vi "主程序-复材超声C扫缺陷分析评定软件.vi"() -> ()   [LabVIEW 2018]
doc: "使用该模板构建用户界面事件处理设计模式。将模板应用于对话框及其它用户界面。用户也可创建并执行VI可按照与用户界面事件相同方式处理的用户定义事件。"
uses:
  <vilib>/Utility/NIReport.llb/Report Type.ctl
  <vilib>/addons/_office/_exclsub.llb/font.ctl
  <vilib>/Utility/NIReport.llb/HTML Report Image Alignment.ctl
  <vilib>/Utility/NIReport.llb/Append Report Text (str wrap).vi
  <vilib>/Utility/NIReport.llb/Append Image to Report (path wrap).vi
  <vilib>/addons/_office/word.llb/Word Easy Table (str).vi
  <vilib>/Utility/NIReport.llb/NI_report.lvclass
  <vilib>/Utility/NIReport.llb/Word/NI_Word.lvclass
  <vilib>/addons/_office/NI_ReportGenerationToolkit.lvlib
  <vilib>/Utility/NIReport.llb/NI_ReportGenerationCore.lvlib
  <vilib>/vision/NI_Vision_Development_Module.lvlib
panel:
  out "框号-报告图中按顺序的值":i32
  out "框号-更新后按顺序的值":i32
  out "XY向分辨率":T1
  out "flag数组":i8[](array[numeric])
  out "字符串":string
  out "图像Y向分辨率（mm/像素）":dbl
  out "图像X向分辨率（mm/像素）":dbl
  out "判定为筋条的长宽比阈值":i32
  out "框号字体大小-":i16
  out "是否需要预处理":u16
  out "计入缺陷的Z值阈值":i32 caption="值"
  out "计入缺陷的面积阈值":i32
  out "报告模式":string
  in  "删除标注":bool caption="定量分析"
  out "缺陷灰度阈值":dbl caption="值"
  out "穿透图原始路径":path
  out "ROImask":T2(plugin-control)
  out "添加的路径":path
  out "连接的字符串 2":string
  out "临界面积百分比值":dbl
  out "临界Z值":i32
  out "标注后的图片路径":path
  out "全部检测结果合并":string[][](table)
  out "全部检测结果":string[][](table)
  out "部位信息":string[](array[string])=["", "34.500000", "32.500000", "1121", "34", "54.955926", "分层类", "不合格", ""]
  in  "完成标注":bool caption="定量分析"
  out "框数":dbl
  out "自定义字体":T3={"Desired Font (Application)"=enum."Application Font", "[User-specified Font]"={"Font Name"="", "Size"=12, "Strikeout?"=FALSE, "Italic?"=FALSE, "Underline?"=FALSE, "Outline?"=FALSE, "Shadow?"=FALSE, "Bold?"=FALSE, "Rotation Angle"=0.0}, "Horizontal Alignment"=0, "Vertical Alignment"=0} {"Horizontal Alignment" items=["Left", "Center", "Right"]; "Vertical Alignment" items=["Bottom", "Top", "Baseline"]}
  out "框组":T4(array[cluster])
  out "质量等级":string
  in  "stop":bool caption="停止"
  in  "导入图像":bool caption="导入图片"
  in  "开始标注":bool caption="定量分析"
  in  "查看评定结果":bool caption="辅助定性分析"
  in  "生成报告":bool caption="生成原始记录"
  in  "控件":enum32{"穿透图"}(tab)
  out "穿透图":T2(plugin-control)
  out "产品规格":cluster{"产品长度（周长）（mm）":dbl, "产品宽度（母线长）（mm）":dbl}
  out "图像分辨率":T1
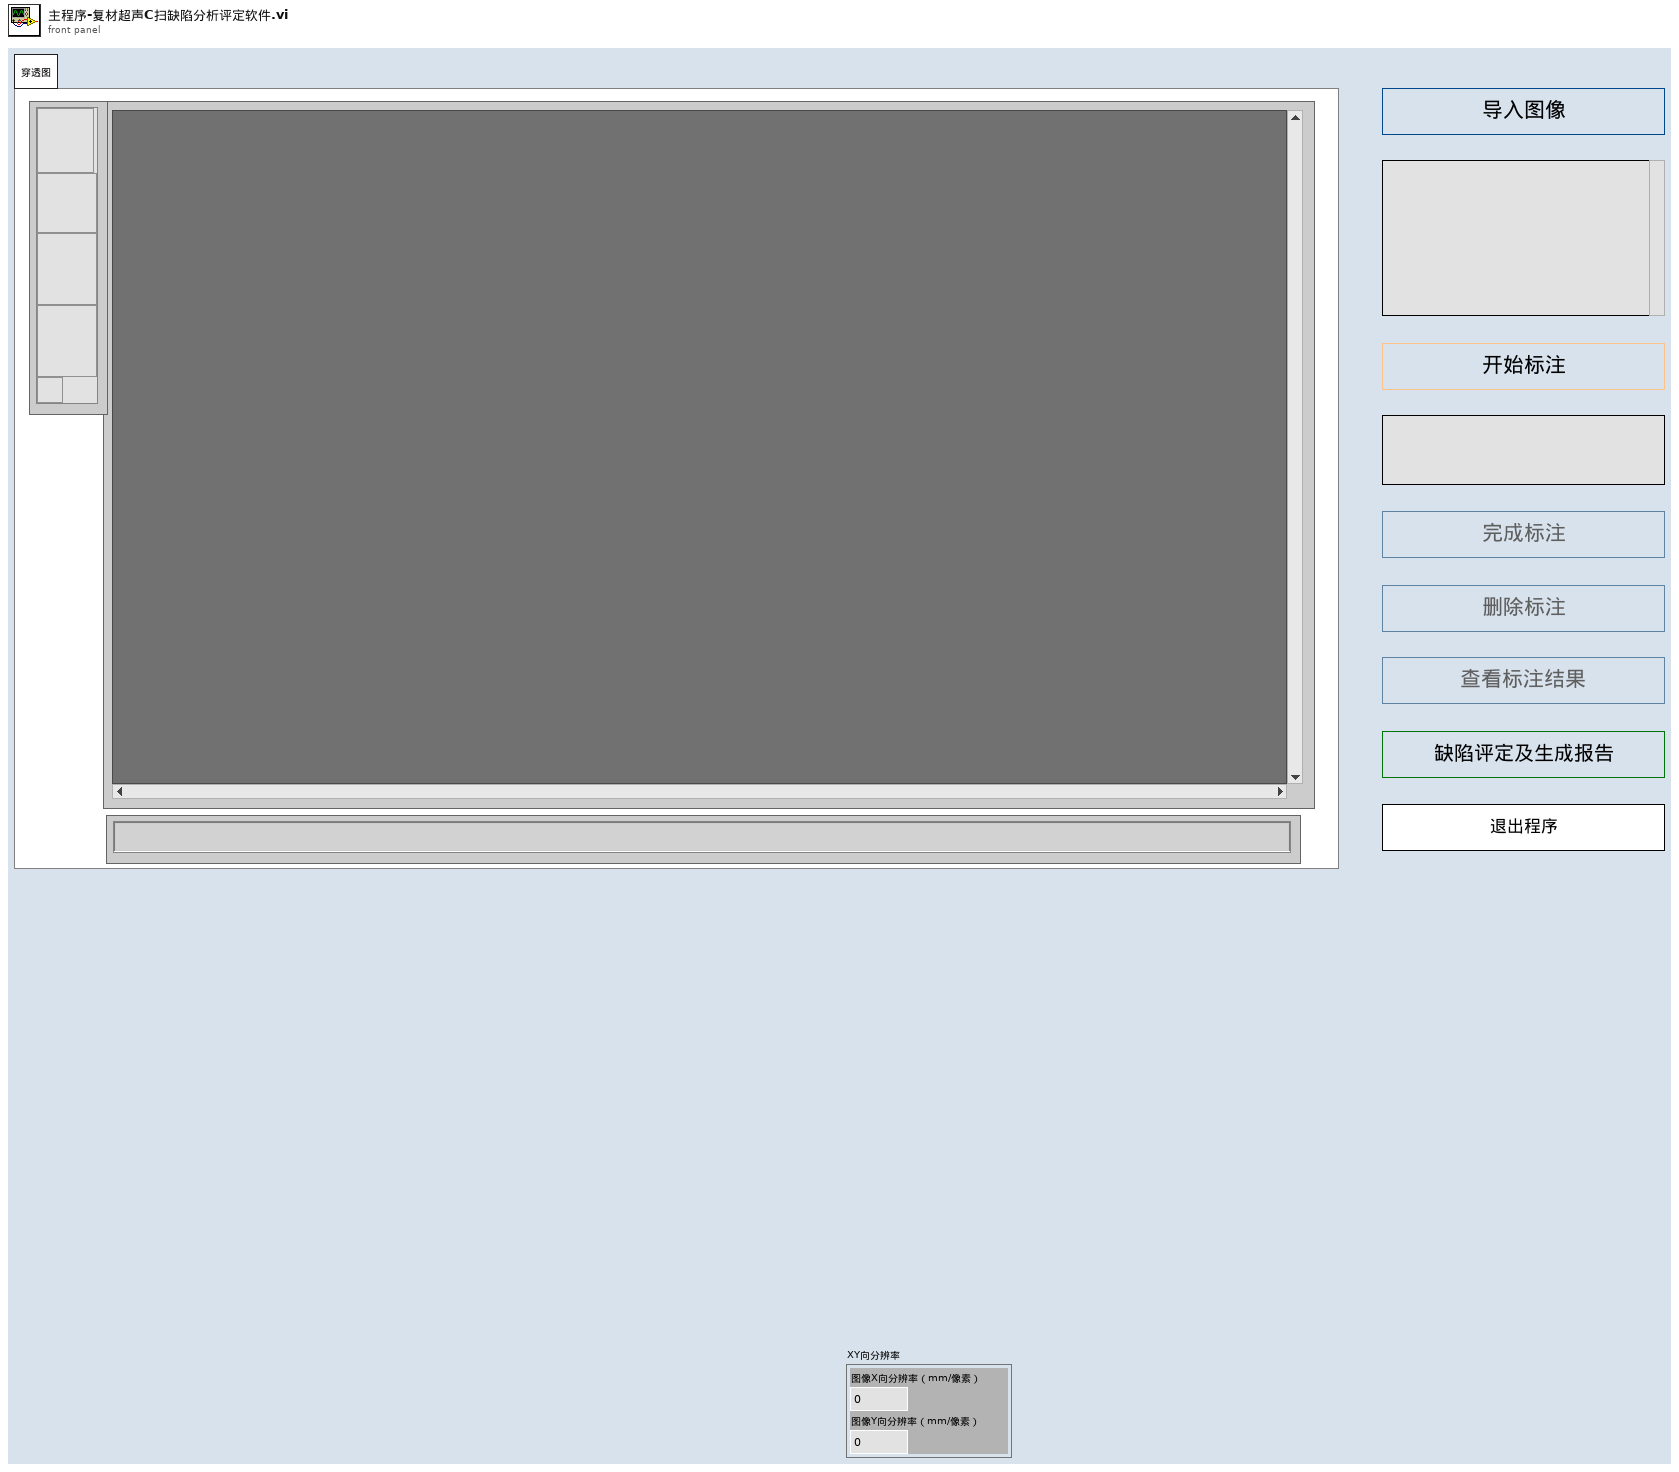
[diagram p1: front panel]
types:
  T1 = cluster{"图像X向分辨率（mm/像素）":dbl, "图像Y向分辨率（mm/像素）":dbl}
  T2 = typedef "IMAQ Image.ctl" = refnum<image>
  T3 = cluster{"Desired Font (Application)":enum16{"User-specified Font", "Application Font", "System Font", "Dialog Font"}, "[User-specified Font]":cluster{"Font Name":string, "Size":i16, "Strikeout?":bool, "Italic?":bool, "Underline?":bool, "Outline?":bool, "Shadow?":bool, "Bold?":bool, "Rotation Angle":dbl}, "Horizontal Alignment":i16, "Vertical Alignment":i16}
  T4 = cluster{"Global Rectangle":i32[], "Contours":cluster{"Contour Type":u32, "ROI Type":u32, "Points":i32[]}[]}[]
  T5 = enum8{"Enabled", "Disabled", "Disabled and Grayed Out"}
  T6 = cluster{"Global Rectangle":i32[], "Contours":cluster{"Contour Type":u32, "ROI Type":u32, "Points":i32[]}[]}
  T7 = cluster{"Zoom Tool":bool, "Selection Tool":bool, "Pan Tool":bool, "Point Tool":bool, "Line Tool":bool, "Rectangle Tool":bool, "Rotated Rectangle Tool":bool, "Polyline Tool":bool, "Polygon Tool":bool, "Freehand Tool":bool, "Closed Freehand Tool":bool, "Ellipse Tool":bool, "Annulus Tool":bool}
  T8 = enum16{"maximized", "minimized", "normal", "no change"}
  T9 = typedef "NI_ReportGenerationCore.lvlib/Report Type.ctl" = enum16{"HTML", "Word", "Excel"}
  T10 = typedef "NI_ReportGenerationCore.lvlib/HTML Report Image Alignment.ctl" = enum16{"(default)", "LEFT", "RIGHT", "TOP", "TEXTTOP", "MIDDLE", "ABSMIDDLE", "BASELINE", "BOTTOM", "ABSBOTTOM"}
  T11 = cluster{"position (Excel)":cluster{"row":i32, "column":i32}, "name (Excel)":string, "bookmark (Word)":string}
  T12 = cluster{"position (excel)":cluster{"row":i32, "column":i32}, "name (excel)":string, "bookmark (word)":string}
  T13 = typedef "NI_ReportGenerationToolkit.lvlib/font.ctl" = cluster{"font name":string, "font size":dbl, "bold":u16, "italic":u16, "underline":u16, "strike through":u16, "font color":u32}
  T14 = typedef "Image Type" = u32
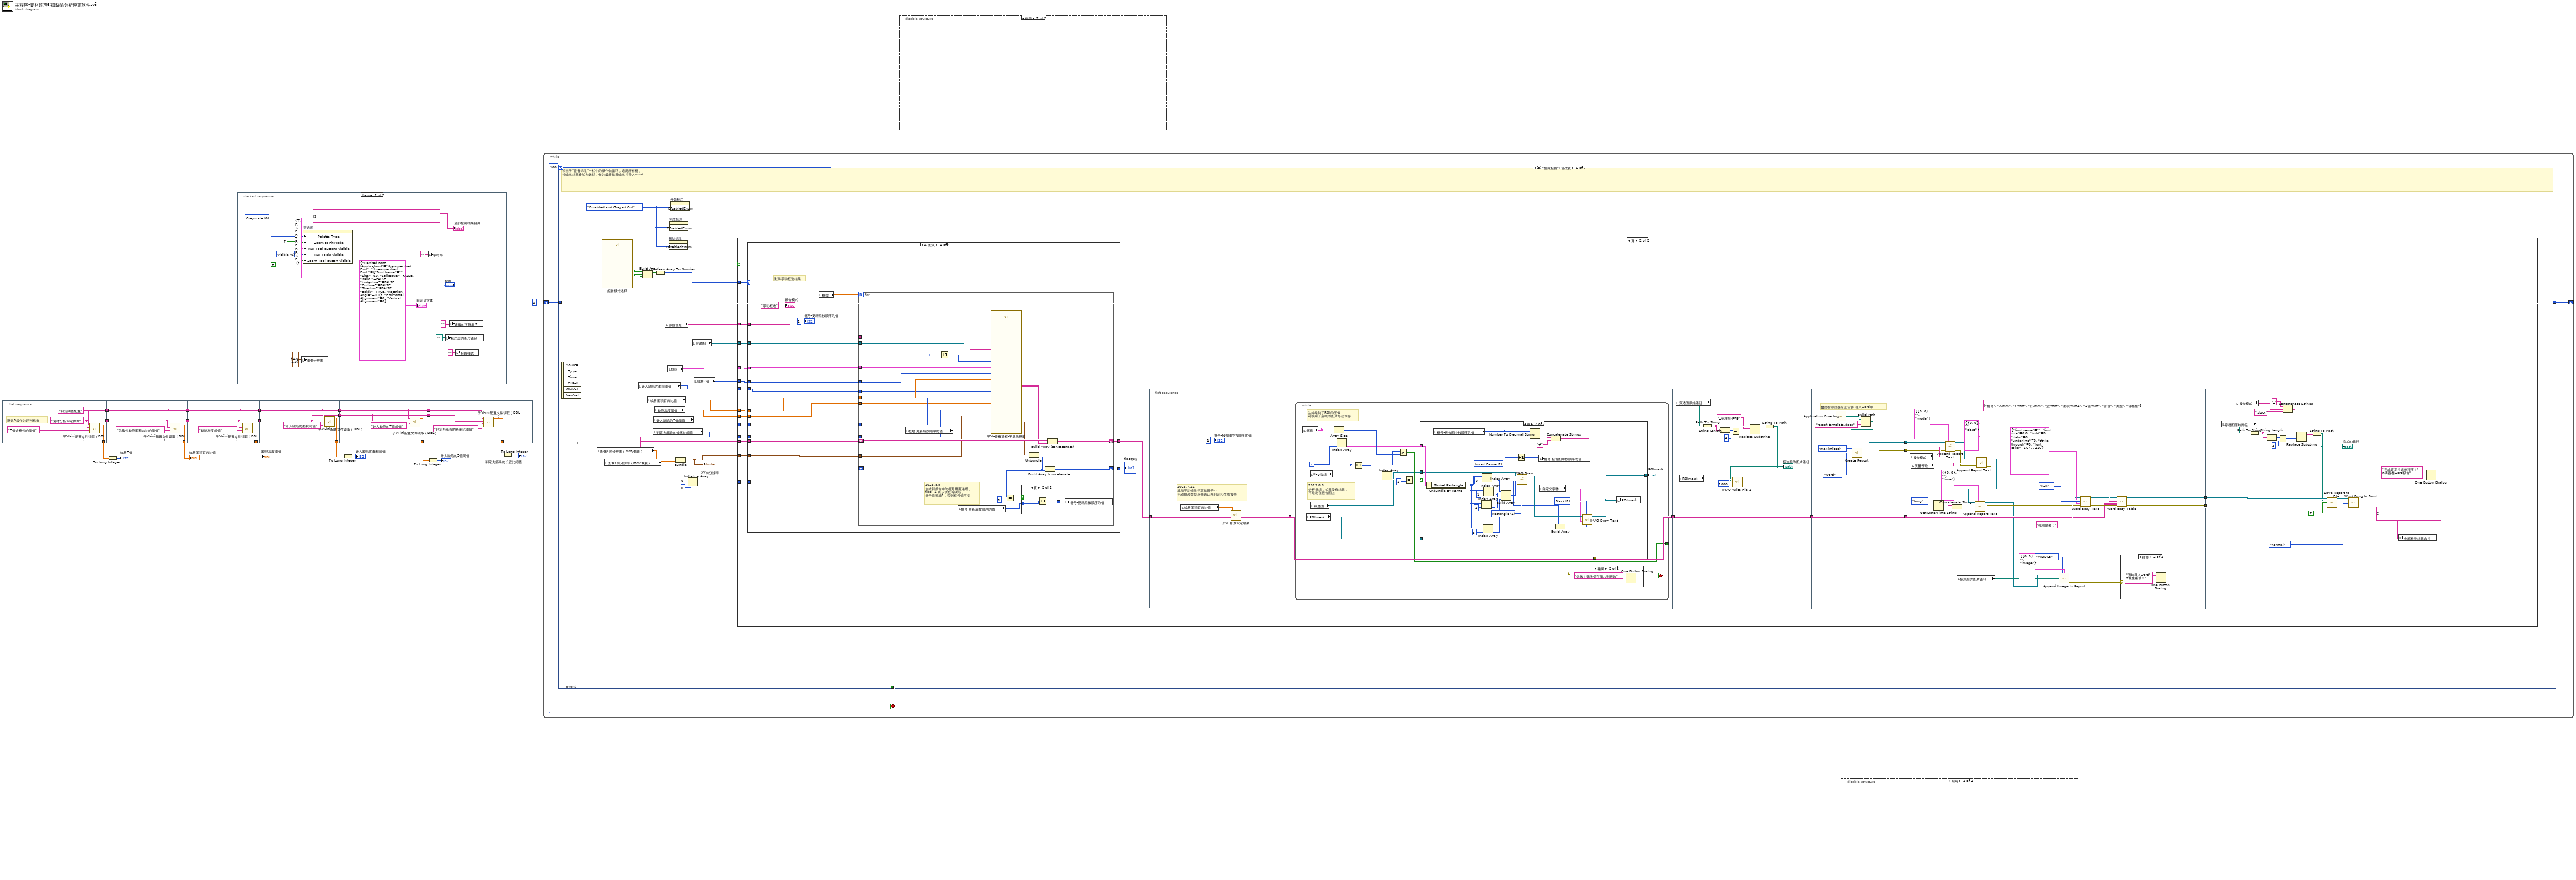
[diagram p0: block diagram]
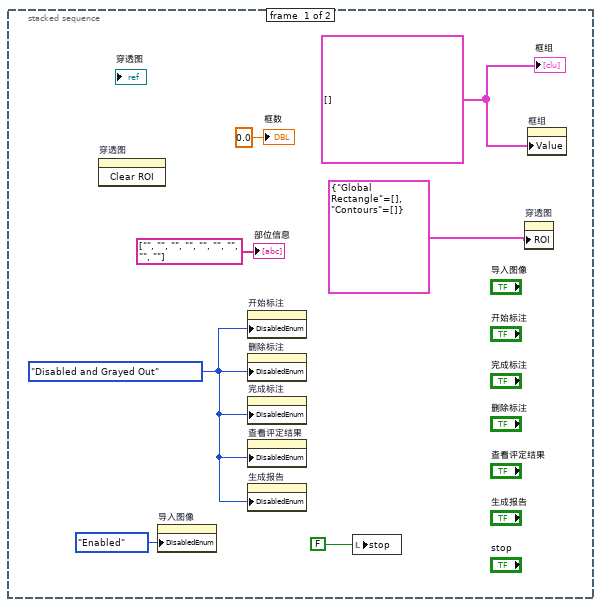
[diagram p3: hidden frame]
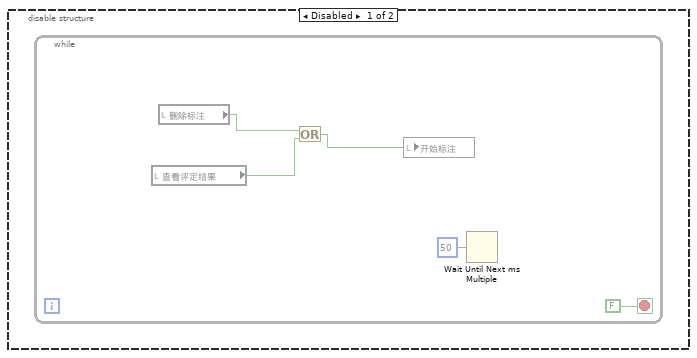
[diagram p4: hidden frame]
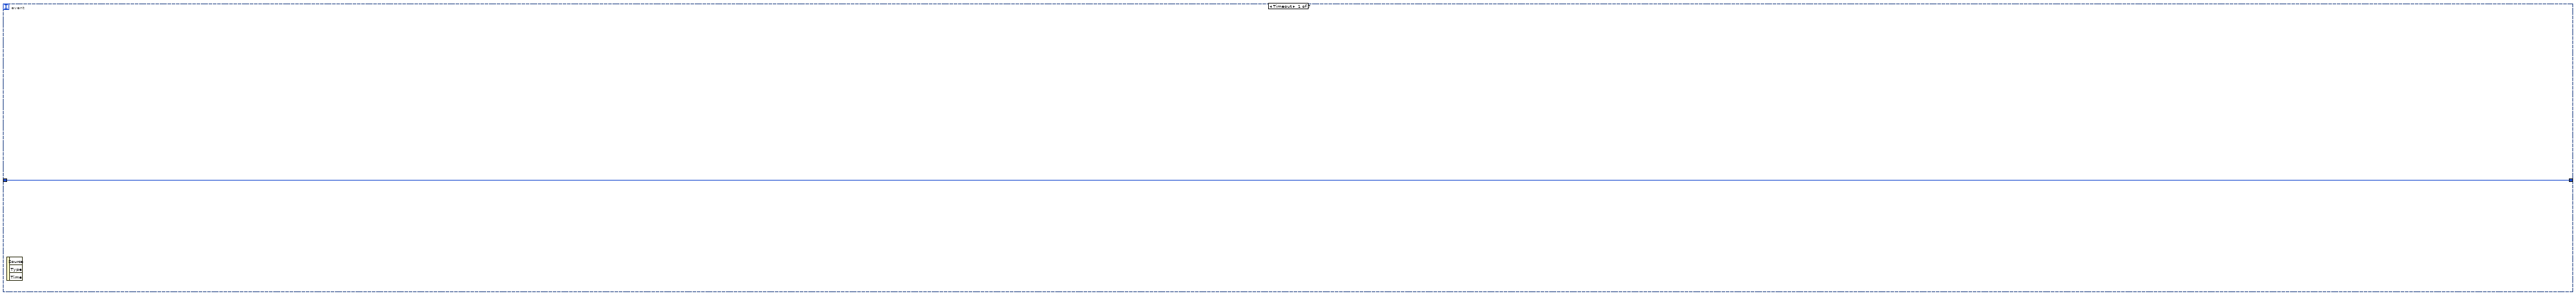
[diagram p5: hidden frame]
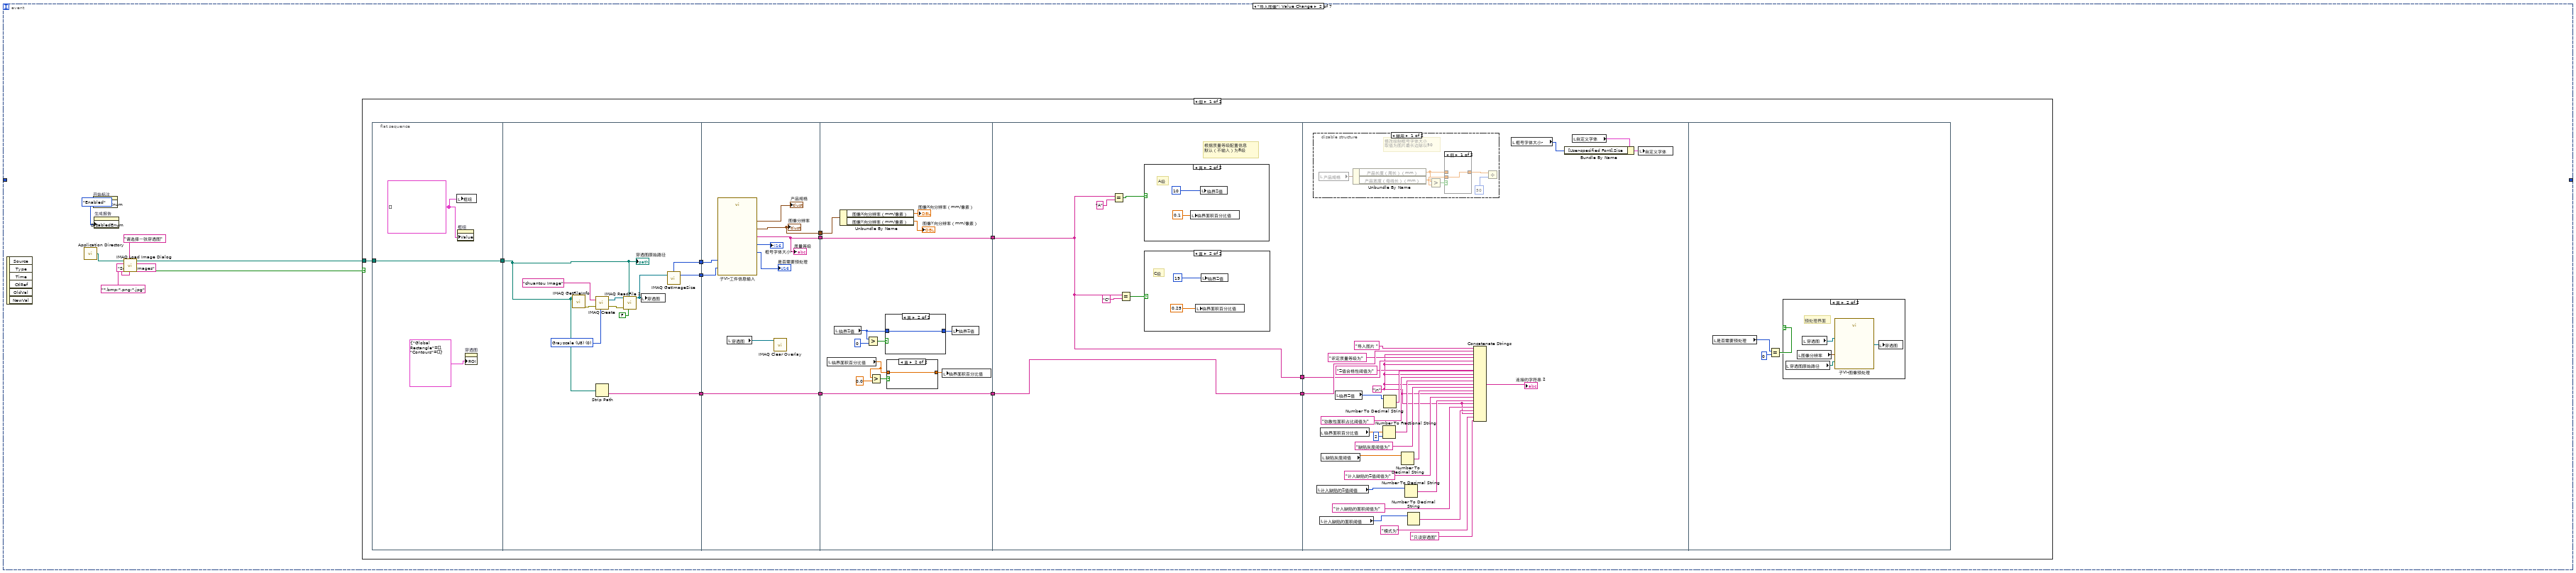
[diagram p6: hidden frame]
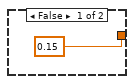
[diagram p7: hidden frame]
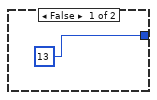
[diagram p8: hidden frame]
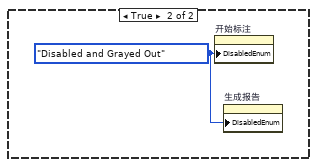
[diagram p14: hidden frame]
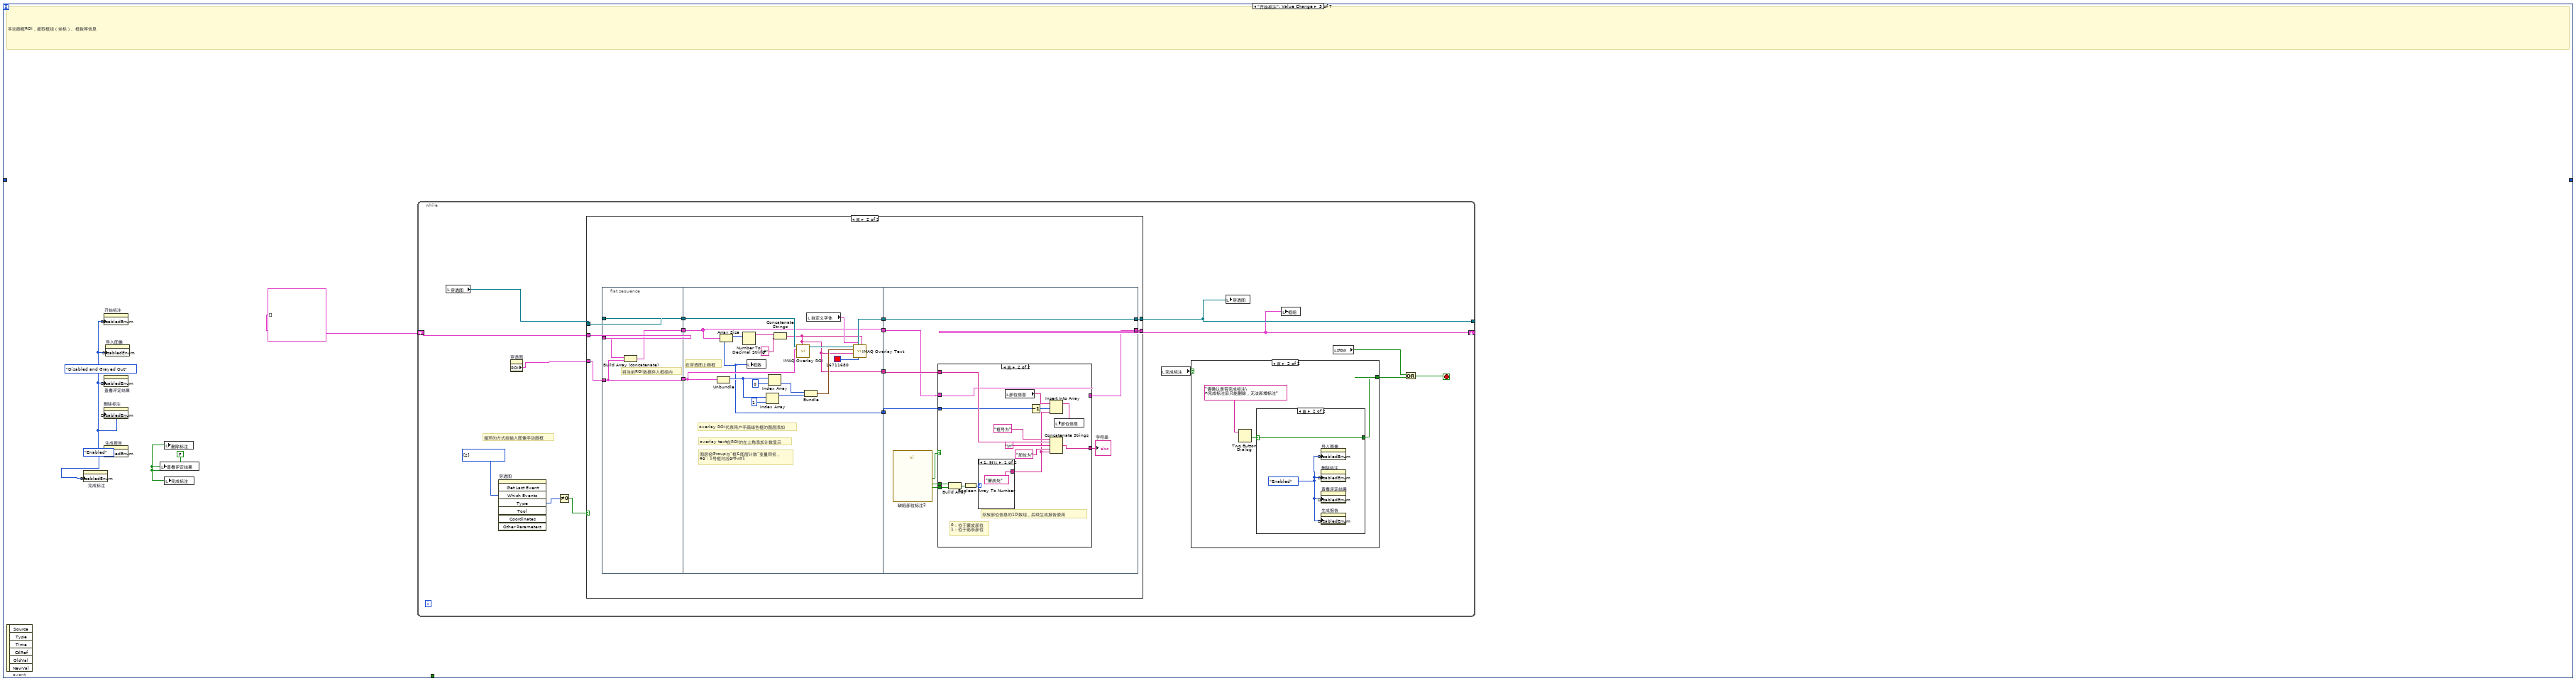
[diagram p15: hidden frame]
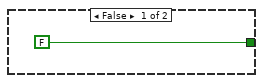
[diagram p16: hidden frame]
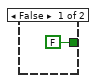
[diagram p17: hidden frame]
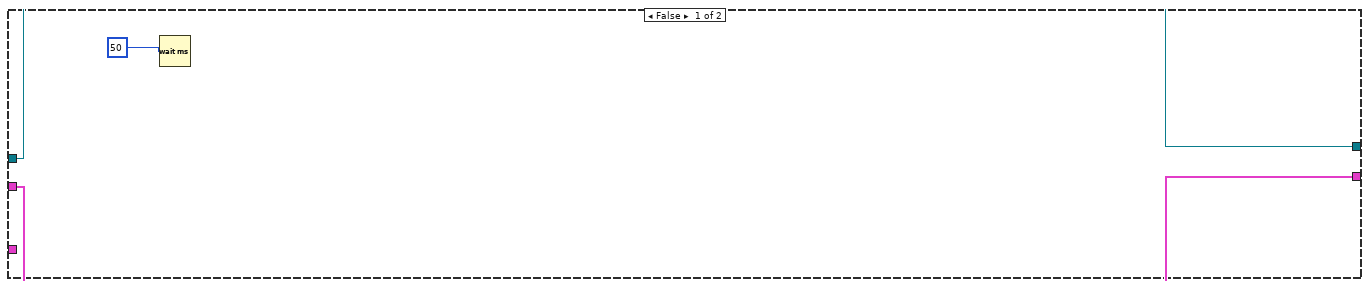
[diagram p18: hidden frame]
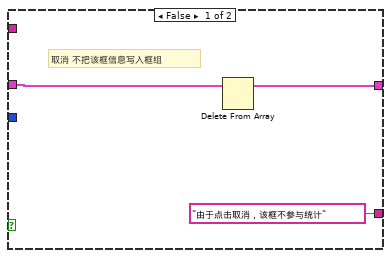
[diagram p19: hidden frame]
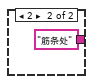
[diagram p20: hidden frame]
diagram:
  n1 = flat-sequence {
    tunnel: [w24] -> w20
    tunnel: [w23] -> w19
    tunnel: [w22] -> w14
    tunnel: w20 -> [w27]
    tunnel: w19 -> [w28]
    tunnel: [w28] -> w18
    tunnel: [w27] -> w17
    tunnel: [w26] -> w15
    tunnel: w18 -> [w30]
    tunnel: w17 -> [w31]
    tunnel: [w32] -> w16
    tunnel: [w31] -> w12
    tunnel: [w30] -> w11
    tunnel: w12 -> [w35]
    tunnel: w11 -> [w34]
    tunnel: [w36] -> w9
    tunnel: [w35] -> w8
    tunnel: [w34] -> w7
    tunnel: w8 -> [w39]
    tunnel: w7 -> [w38]
    tunnel: [w40] -> w5
    tunnel: [w39] -> w4
    tunnel: [w38] -> w3
    tunnel: w4 -> [w45]
    tunnel: w3 -> [w44]
    tunnel: [w42] -> w2
    frame #0 {
      w23 = "复材分析评定软件" ("section")
      w24 = "判定阈值配置" ("文件名称")
      # "默认B级作为评判标准"
      n2 = call "子VI-ini配置文件读取（DBL）.vi"("key"="Z值合格性的阈值", "section"=w23, "文件名称"=w24) -> ("value"=w22:dbl)  [unwired: 8 in]
    }
    frame #1 {
      n3 = call "子VI-ini配置文件读取（DBL）.vi"("key"="弥散性缺陷面积占比的阈值", "section"=w28, "文件名称"=w27) -> ("value"=w26:dbl)  [unwired: 8 in]
    }
    frame #2 {
      n4 = call "子VI-ini配置文件读取（DBL）.vi"("key"="缺陷灰度阈值", "section"=w30, "文件名称"=w31) -> ("value"=w32:dbl)  [unwired: 8 in]
    }
    frame #3 {
      n5 = call "子VI-ini配置文件读取（DBL）.vi"("key"="计入缺陷的面积阈值", "section"=w34, "文件名称"=w35) -> ("value"=w36:dbl)  [unwired: 8 in]
    }
    frame #4 {
      n6 = call "子VI-ini配置文件读取（DBL）.vi"("key"="计入缺陷的Z值阈值", "section"=w38, "文件名称"=w39) -> ("value"=w40:dbl)  [unwired: 8 in]
    }
    frame #5 {
      n7 = call "子VI-ini配置文件读取（DBL）.vi"("key"="判定为筋条的长宽比阈值", "section"=w44, "文件名称"=w45) -> ("value"=w42:dbl)  [unwired: 8 in]
    }
  }
  n8 = To Long Integer(number=w14) -> (32bit integer=→"临界Z值":i32)
  n9 = stacked-sequence {
    frame #0 {
      w50 = T4 [] ("框组")
      w48 = T5."Disabled and Grayed Out" ("禁用")
      n10 = invoke on="穿透图" class="ImageControl" method="Clear ROI"() -> ()  [unwired: 3 in, 3 out]
      n11 = property on="导入图像" class="Bool"("DisabledEnum"=T5."Enabled" ("禁用")) -> ()  [unwired: 2 in, 2 out]
      n12 = property on="开始标注" class="Bool"("DisabledEnum"=w48) -> ()  [unwired: 2 in, 2 out]
      n13 = property on="删除标注" class="Bool (严格)"("DisabledEnum"=w48) -> ()  [unwired: 2 in, 2 out]
      n14 = property on="完成标注" class="Bool (严格)"("DisabledEnum"=w48) -> ()  [unwired: 2 in, 2 out]
      n15 = property on="查看评定结果" class="Bool (严格)"("DisabledEnum"=w48) -> ()  [unwired: 2 in, 2 out]
      n16 = property on="生成报告" class="Bool"("DisabledEnum"=w48) -> ()  [unwired: 2 in, 2 out]
      n17 = local write "stop"(FALSE ("stop")) -> ()
      n18 = property on="穿透图" class="ImageControl"("ROI"=T6 {"Global Rectangle"=[], "Contours"=[]}) -> ()  [unwired: 2 in, 2 out]
      n19 = property on="框组" class="Arr (严格)"("Value"=w50) -> ()  [unwired: 2 in, 2 out]
      "部位信息" <- string[] ["", "", "", "", "", "", "", "", ""] ("部位信息")
      "框组" <- w50
      "框数" <- 0.0 ("框数")
    }
    frame #1 {
      w54 = u32 0 items=["Visible", "Hidden", "Hidden, Use WindTools Palette"] ("ROI Tools Visible")
      w57 = u32 0 items=["Grayscale", "Binary", "Gradient", "Rainbow", "Temperature", "User Defined", "Binary 16 Bit", "Gradient 16 Bit", "Rainbow 16 Bit", "Temperature 16 Bit", "User Defined 16 Bit"] ("Palette:Palette Type")
      n20 = local write "图像分辨率"(T1 {"图像X向分辨率（mm/像素）"=1.0, "图像Y向分辨率（mm/像素）"=1.0} ("图像分辨率")) -> ()
      n21 = property on="穿透图" class="ImageControl"("Palette Type"=w57, "Zoom to Fit Mode"=TRUE, "ROI Tool Buttons Visible"=T7 {"Zoom Tool"=TRUE, "Selection Tool"=FALSE, "Pan Tool"=TRUE, "Point Tool"=FALSE, "Line Tool"=FALSE, "Rectangle Tool"=TRUE, "Rotated Rectangle Tool"=FALSE, "Polyline Tool"=FALSE, "Polygon Tool"=FALSE, "Freehand Tool"=FALSE, "Closed Freehand Tool"=TRUE, "Ellipse Tool"=FALSE, "Annulus Tool"=TRUE} ("ROI Tool Buttons Visible:All Elements"), "ROI Tools Visible"=w54, "Zoom Tool Button Visible"=TRUE ("ROI Tool Buttons Visible:Zoom Tool Button Visible")) -> ()  [unwired: 2 in, 2 out]
      n22 = local write "字符串"("" ("字符串")) -> ()
      n23 = local write "标注后的图片路径"(path "" ("标注后的图片路径")) -> ()
      n24 = local write "连接的字符串 2"("" ("连接的字符串 2")) -> ()
      n25 = local write "报告模式"("" ("报告模式")) -> ()
      "自定义字体" <- T3 {"Desired Font (Application)"=enum."User-specified Font", "[User-specified Font]"={"Font Name"="", "Size"=60, "Strikeout?"=FALSE, "Italic?"=FALSE, "Underline?"=FALSE, "Outline?"=FALSE, "Shadow?"=FALSE, "Bold?"=TRUE, "Rotation Angle"=0.0}, "Horizontal Alignment"=0, "Vertical Alignment"=0} ("Font, Size & Style")
      "全部检测结果合并" <- string[][] [] ("弥散类检测结果合并")
    }
  }
  n26 = To Long Integer(number=w9) -> (32bit integer=→"计入缺陷的面积阈值":i32)
  n27 = To Long Integer(number=w5) -> (32bit integer=→"计入缺陷的Z值阈值":i32)
  n28 = To Long Integer(number=w2) -> (32bit integer=→"判定为筋条的长宽比阈值":i32)
  n29 = while {
    shift-right: [w65] -> _
    shift-left: 0 -> [w66]
    stop <- w68 stop-if-true
    n30 = event shown="[5] \"生成报告\": 值改变" {
      selector: _ -> [_ _ _ _ _ _ _]
      dyn-events: _ -> [_ _ _ _ _ _ _]
      timeout: 100 -> [_ _ _ _ _ _ _]
      tunnel: [_ _ _ _ _ _ w600] -> w68
      tunnel: w66 -> [w69 _ _ _ _ w340 _]
      tunnel: [w69 _ _ _ _ w340 0] -> w65
      event Timeout {
        n31 = event-data() -> ()  [unwired: 1 in, 3 out]
      }
      event "导入图像": Value Change {
        w71 = T5."Enabled" ("禁用")
        n32 = event-data() -> ()  [unwired: 1 in, 6 out]
        n33 = call <vilib>:"Application Directory.vi"() -> ("Application Directory"=w70:path)
        n34 = property on="开始标注" class="Bool"("DisabledEnum"=w71) -> ()  [unwired: 2 in, 2 out]
        n35 = property on="生成报告" class="Bool"("DisabledEnum"=w71) -> ()  [unwired: 2 in, 2 out]
        n36 = call "IMAQ Load Image Dialog"("Pattern Label"="Source Images", "Prompt"="请选择一张穿透图" ("prompt"), "Pattern"="*.bmp;*.png;*.jpg", "Start Path"=w70) -> ("Cancelled?"=w73:bool, "Path"=w72:path)  [unwired: 5 in, 1 out]
        n37 = case shown="假" w73 {
          tunnel: w72 -> [w86 _]
          frame False {
            n38 = flat-sequence {
              tunnel: w86 -> [w90]
              tunnel: [w90] -> w85
              tunnel: w85 -> [w93]
              tunnel: [w95] -> w84
              tunnel: [w94] -> w83
              tunnel: [w92] -> w82
              tunnel: [w110] -> w88
              tunnel: w84 -> [w109]
              tunnel: w83 -> [w108]
              tunnel: w82 -> [w107]
              tunnel: [w107] -> w81
              tunnel: [w103] -> w77
              tunnel: w88 -> [w124]
              tunnel: [w124] -> w87
              tunnel: w81 -> [w123]
              tunnel: [w123] -> w80
              tunnel: w77 -> [w114]
              tunnel: w87 -> [w129]
              tunnel: w80 -> [w130]
              tunnel: [w130] -> w79
              tunnel: [w129] -> w78
              tunnel: w79 -> [w156]
              tunnel: w78 -> [w154]
              frame #0 {
                w91 = T4 [] ("框组")
                n39 = local write "框组"(w91) -> ()
                n40 = property on="框组" class="Arr (严格)"("Value"=w91) -> ()  [unwired: 2 in, 2 out]
                n41 = property on="穿透图" class="ImageControl"("ROI"=T6 {"Global Rectangle"=[], "Contours"=[]}) -> ()  [unwired: 2 in, 2 out]
              }
              frame #1 {
                w97 = T14 0 items=["Grayscale (U8)", "Grayscale (I16)", "Grayscale (SGL)", "Complex (CSG)", "RGB (U32)", "HSL (U32)", "RGB (U64)", "Grayscale (U16)"] ("Image Type")
                n42 = call "IMAQ GetFileInfo"("File Path"=w93) -> ("error out"=w100:errorcluster)  [unwired: 4 in, 6 out]
                n43 = call "IMAQ Create"("Image Name"="chuantou Image", "Image Type"=w97, "error in (no error)"=w100) -> ("New Image"=w101:T2, "error out"=w102:errorcluster)  [unwired: 2 in]
                n44 = Strip Path(path=w93) -> (name=w92:string)  [unwired: 1 out]
                n45 = call "IMAQ ReadFile 2"("Use File Path Image Type"=FALSE, "File Path"=w93, "error in (no error)"=w102, "Image"=w101) -> ("Image Out"=w99:T2)  [unwired: 3 in, 4 out]
                n46 = local write "穿透图"(w99) -> ()
                n47 = call "IMAQ GetImageSize"("Image"=w99) -> ("Y Resolution"=w94:i32, "X Resolution"=w95:i32)  [unwired: 3 in, 1 out]
                "穿透图原始路径" <- w93
              }
              frame #2 {
                n48 = call "子VI-工件信息输入.vi"("Y Resolution"=w108, "X Resolution"=w109) -> ("质量等级"=w110:string, "框号字体大小-"=→"框号字体大小-":i16, "产品规格"=→"产品规格":cluster{"产品长度（周长）（mm）":dbl, "产品宽度（母线长）（mm）":dbl}, "是否需要预处理"=→"是否需要预处理":u16, "图像分辨率"=w103:T1)  [unwired: 5 in]
                "图像分辨率" <- w103
                "质量等级" <- w110
                n49 = local read "穿透图"() -> (w106:T2)
                n50 = call "IMAQ Clear Overlay"("Image"=w106) -> ()  [unwired: 9 in, 2 out]
              }
              frame #3 {
                n51 = local read "临界面积百分比值"() -> (w115:dbl)
                n52 = local read "临界Z值"() -> (w116:i32)
                n53 = Unbundle By Name(w114) -> ("图像X向分辨率（mm/像素）"=→"图像X向分辨率（mm/像素）":dbl, "图像Y向分辨率（mm/像素）"=→"图像Y向分辨率（mm/像素）":dbl)
                n54 = Greater?(x=w116, y=0) -> (0:w121:bool)
                n55 = Greater?(x=w115, y=0.0) -> (0:w119:bool)
                n56 = case shown="真" w121 {
                  tunnel: [13 ("临界Z值") w128] -> w118
                  tunnel: w116 -> [_ w128]
                  frame False {
                  }
                  frame True {
                  }
                }
                n57 = case shown="真" w119 {
                  tunnel: [0.15 ("临界面积百分比值") w126] -> w117
                  tunnel: w115 -> [_ w126]
                  frame False {
                  }
                  frame True {
                  }
                }
                n58 = local write "临界面积百分比值"(w117) -> ()
                n59 = local write "临界Z值"(w118) -> ()
              }
              frame #4 {
                # "根据质量等级配置信息\n默认（不输入）为B级"
                n60 = Equal?(x=w129, y="A") -> (x = y?=w133:bool)
                n61 = Equal?(x=w129, y="C") -> (x = y?=w134:bool)
                n62 = case shown="真" w133 {
                  frame False {
                  }
                  frame True {
                    # "A级"
                    n63 = local write "临界面积百分比值"(0.1 ("临界面积百分比值")) -> ()
                    n64 = local write "临界Z值"(10 ("临界Z值")) -> ()
                  }
                }
                n65 = case shown="真" w134 {
                  frame False {
                  }
                  frame True {
                    # "C级"
                    n66 = local write "临界面积百分比值"(0.25 ("临界面积百分比值")) -> ()
                    n67 = local write "临界Z值"(19 ("临界Z值")) -> ()
                  }
                }
              }
              frame #5 {
                w144 = "\n"
                n68 = disable-structure shown="禁用" {
                  frame Disabled {
                    # "修改绘制框号字体大小\n取值为图片最长边除以50"
                    n69 = local read "产品规格"() -> (w167:cluster{"产品长度（周长）（mm）":dbl, "产品宽度（母线长）（mm）":dbl})
                    n70 = Unbundle By Name(w167) -> ("产品长度（周长）（mm）"=w169:dbl, "产品宽度（母线长）（mm）"=w170:dbl)
                    n71 = Greater?(x=w169, y=w170) -> (0:w168:bool)
                    n72 = case shown="假" w168 {
                      tunnel: w169 -> [_ w173]
                      tunnel: w170 -> [w172 _]
                      tunnel: [w172 w173] -> w171
                      frame False {
                      }
                      frame True {
                      }
                    }
                    n73 = Divide(x=w171, y=i8 50) -> ()  [unwired: 1 out]
                  }
                  frame Enabled {
                  }
                }
                n74 = local read "计入缺陷的Z值阈值"() -> (w150:i32)
                n75 = local read "计入缺陷的面积阈值"() -> (w147:i32)
                n76 = local read "临界面积百分比值"() -> (w162:dbl)
                n77 = local read "缺陷灰度阈值"() -> (w164:dbl)
                n78 = local read "临界Z值"() -> (w160:i32)
                n79 = Number To Fractional String(number=w162, precision (6)=i16 2 ("精度(6)")) -> (F-format string=w163:string)  [unwired: 2 in]
                n80 = Number To Decimal String(number=w160) -> (decimal integer string=w161:string)  [unwired: 1 in]
                n81 = Number To Decimal String(number=w164) -> (decimal integer string=w165:string)  [unwired: 1 in]
                n82 = Number To Decimal String(number=w150) -> (decimal integer string=w148:string)  [unwired: 1 in]
                n83 = Number To Decimal String(number=w147) -> (decimal integer string=w145:string)  [unwired: 1 in]
                n84 = Concatenate Strings("导入图片 " ("字符串"), w156, w144, "评定质量等级为" ("字符串"), w154, w144, "Z值合格性阈值为" ("字符串"), w161, w144, "弥散性面积占比阈值为" ("字符串"), w163, w144, "缺陷灰度阈值为" ("字符串"), w165, w144, "计入缺陷的Z值阈值为" ("字符串"), w148, w144, "计入缺陷的面积阈值为" ("字符串"), w145, w144, "模式为" ("字符串"), "只读穿透图" ("字符串")) -> (→"连接的字符串 2":string)
                n85 = local read "框号字体大小-"() -> (w140:i16)
                n86 = local read "自定义字体"() -> (w141:T3)
                n87 = Bundle By Name(cluster=w141, "[User-specified Font].Size"=w140) -> (w142:T3)
                n88 = local write "自定义字体"(w142) -> ()
              }
              frame #6 {
                n89 = local read "是否需要预处理"() -> (w175:u16)
                n90 = Equal?(x=w175, y=u16 0) -> (x = y?=w176:bool)
                n91 = case shown="真" w176 {
                  frame False {
                  }
                  frame True {
                    # "预处理界面"
                    n92 = local read "穿透图原始路径"() -> (w177:path)
                    n93 = local read "图像分辨率"() -> (w178:T1)
                    n94 = local read "穿透图"() -> (w180:T2)
                    n95 = call "子VI-图像预处理.vi"("图像分辨率"=w178, "穿透图"=w180, "穿透图原始路径"=w177) -> ("穿透图out"=w179:T2)  [unwired: 8 in]
                    n96 = local write "穿透图"(w179) -> ()
                  }
                }
              }
            }
          }
          frame True {
            w181 = T5."Disabled and Grayed Out" ("禁用")
            n97 = property on="开始标注" class="Bool"("DisabledEnum"=w181) -> ()  [unwired: 2 in, 2 out]
            n98 = property on="生成报告" class="Bool"("DisabledEnum"=w181) -> ()  [unwired: 2 in, 2 out]
          }
        }
      }
      event "开始标注": Value Change {
        w183 = T5."Disabled and Grayed Out" ("禁用")
        w185 = FALSE ("完成标注")
        # "手动画框ROI，提取框组（坐标）、框数等信息"
        n99 = event-data() -> ()  [unwired: 1 in, 6 out]
        n100 = property on="完成标注" class="Bool (严格)"("DisabledEnum"=T5."Enabled" ("禁用")) -> ()  [unwired: 2 in, 2 out]
        n101 = property on="查看评定结果" class="Bool (严格)"("DisabledEnum"=w183) -> ()  [unwired: 2 in, 2 out]
        n102 = property on="删除标注" class="Bool (严格)"("DisabledEnum"=w183) -> ()  [unwired: 2 in, 2 out]
        n103 = property on="生成报告" class="Bool"("DisabledEnum"=w183) -> ()  [unwired: 2 in, 2 out]
        n104 = property on="开始标注" class="Bool"("DisabledEnum"=w183) -> ()  [unwired: 2 in, 2 out]
        n105 = property on="导入图像" class="Bool"("DisabledEnum"=w183) -> ()  [unwired: 2 in, 2 out]
        n106 = local write "查看评定结果"(w185) -> ()
        n107 = local write "删除标注"(w185) -> ()
        n108 = local write "完成标注"(w185) -> ()
        n109 = while {
          shift-right: [w190] -> _
          shift-left: T4 [] ("框组") -> [w197]
          tunnel: [w195] -> _
          stop <- w189 stop-if-true
          (unwired) "_" ("名称或相对路径")
          (unwired) ".docx" ("名称或相对路径")
          w188 = i32[] [2] items=["No Event"=0, "Click Event"=1, "Draw Event"=2, "Size Event"=4, "Scroll Event"=5, "Double Click Event"=8] ("Which Events")
          # "循环的方式给输入图像手动画框"
          n110 = local read "穿透图"() -> (w196:T2)
          n111 = invoke on="穿透图" class="ImageControl" method="Get Last Event"("Which Events"=w188) -> ("Type"=w187:i32)  [unwired: 7 in, 7 out]
          n112 = property on="穿透图" class="ImageControl"() -> ("ROI"=w186:T6)  [unwired: 2 in, 2 out]
          n113 = Not Equal To 0?(x=w187) -> (x != 0?=w191:bool)
          n114 = case shown="真" w191 {
            tunnel: w196 -> [w208 w220]
            tunnel: [w208 w219] -> w195
            tunnel: [w206 w217] -> w190
            tunnel: w197 -> [w206 w218]
            tunnel: w186 -> [_ w216]
            frame False {
              n115 = Wait (ms)(milliseconds to wait=u32 50 ("毫秒倍数")) -> ()  [unwired: 1 out]
              n116 = Wait (ms)(milliseconds to wait=u32 50) -> ()  [unwired: 1 out]
            }
            frame True {
              n117 = flat-sequence {
                tunnel: w220 -> [w221]
                tunnel: [w221] -> w215
                tunnel: w216 -> [w224]
                tunnel: [w224] -> w214
                tunnel: w218 -> [w223]
                tunnel: [w222] -> w213
                tunnel: w215 -> [w233]
                tunnel: w214 -> [w232]
                tunnel: w213 -> [w225]
                tunnel: [w235] -> w212
                tunnel: [w225] -> w211
                tunnel: [w229] -> w210
                tunnel: [w227] -> w209
                tunnel: w212 -> [w250]
                tunnel: w211 -> [w244]
                tunnel: w210 -> [w247]
                tunnel: w209 -> [w246]
                tunnel: [w250] -> w219
                tunnel: [w243] -> w217
                frame #0 {
                  # "将当前ROI数据存入框组内"
                  n118 = Build Array (concatenate)(w223, w224) -> (w222:T4)
                }
                frame #1 {
                  # "在穿透图上画框"
                  # "图层名Group与“框&图层计数”变量同名，\neg：1号框对应group1"
                  # "overlay text在ROI的左上角添加计数显示"
                  # "overlay ROI代表用户手画绿色框的图层添加"
                  n119 = Unbundle(w232) -> ("Global Rectangle"=w240:i32[])  [unwired: 1 out]
                  n120 = Array Size(array=w225) -> (size(s)=w227:i32)
                  n121 = Number To Decimal String(number=w227) -> (decimal integer string=w228:string)  [unwired: 1 in]
                  n122 = local write "框数"(w227) -> ()
                  n123 = Index Array(array=w240, index=1 ("索引")) -> (element=w238:i32)
                  n124 = Index Array(array=w240, index=0 ("索引")) -> (element=w239:i32)
                  n125 = Concatenate Strings(w228, "#" ("字符串")) -> (w229:string)
                  n126 = call "IMAQ Overlay ROI"("Group"=w229, "ROI Descriptor"=w232, "Image"=w233) -> ("Image Out"=w241:T2)  [unwired: 7 in, 1 out]
                  n127 = Bundle(w239, w238) -> (w234:cluster{i32, i32})  [unwired: 1 in]
                  n128 = local read "自定义字体"() -> (w231:T3)
                  n129 = call "IMAQ Overlay Text"("Group"=w229, "Text Color (black)"=u32 16711680, "Font, Size & Style"=w231, "String"=w229, "Origin"=w234, "Image"=w241) -> ("Image Out"=w235:T2)  [unwired: 4 in, 1 out]
                }
                frame #2 {
                  n130 = call "缺陷部位标注2"() -> ("位于筋条处"=w249:bool, "位于蒙皮处"=w248:bool, "确定"=w245:bool)  [unwired: 16 in, 1 out]
                  n131 = case shown="真" w245 {
                    tunnel: w249 -> [_ w266]
                    tunnel: w248 -> [_ w265]
                    tunnel: w247 -> [_ w261]
                    tunnel: w246 -> [_ w258]
                    tunnel: w244 -> [w253 w255]
                    tunnel: [w252 w255] -> w243
                    tunnel: ["由于点击取消，该框不参与统计" w254] -> w242
                    frame False {
                      # "取消 不把该框信息写入框组"
                      n132 = Delete From Array(array=w253) -> (array with subset deleted=w252:T4)  [unwired: 2 in, 1 out]
                    }
                    frame True {
                      # "0：位于蒙皮部位\n1：位于筋条部位"
                      # "存放部位信息的1D数组，后续生成报告使用"
                      n133 = Build Array(w265, w266) -> (w267:bool[])
                      n134 = Boolean Array To Number(Boolean array=w267) -> (number=w268:u32)
                      n135 = case shown="1, 默认" w268 {
                        tunnel: ["蒙皮处" ("t") "筋条处" ("t")] -> w256
                        frame 1, Default {
                        }
                        frame 2 {
                        }
                      }
                      n136 = local read "部位信息"() -> (w260:string[])
                      n137 = Decrement(x=w258) -> (x-1=w257:i32)
                      n138 = Insert Into Array(array=w260, index=w257, new element=w256) -> (w259:string[])
                      n139 = Concatenate Strings("框号为" ("字符串"), w261, "\n", "部位为" ("字符串"), w256) -> (w254:string)
                      n140 = local write "部位信息"(w259) -> ()
                    }
                  }
                  "字符串" <- w242
                }
              }
            }
          }
          n141 = local read "完成标注"() -> (w193:bool)
          n142 = case shown="真" w193 {
            tunnel: [FALSE ("T button?") w199] -> w192
            frame False {
            }
            frame True {
              n143 = Two Button Dialog(message="请确认是否完成标注\n完成标注后只能删除，无法新增标注" ("消息")) -> (T button?=w200:bool)  [unwired: 2 in]
              n144 = case shown="真" w200 {
                selector: w200 -> [_ w204]
                tunnel: [FALSE w204] -> w199
                frame False {
                }
                frame True {
                  w203 = T5."Enabled" ("禁用")
                  n145 = property on="导入图像" class="Bool"("DisabledEnum"=w203) -> ()  [unwired: 2 in, 2 out]
                  n146 = property on="删除标注" class="Bool (严格)"("DisabledEnum"=w203) -> ()  [unwired: 2 in, 2 out]
                  n147 = property on="查看评定结果" class="Bool (严格)"("DisabledEnum"=w203) -> ()  [unwired: 2 in, 2 out]
                  n148 = property on="生成报告" class="Bool"("DisabledEnum"=w203) -> ()  [unwired: 2 in, 2 out]
                }
              }
            }
          }
          n149 = local write "穿透图"(w195) -> ()
          n150 = local write "框组"(w190) -> ()
          n151 = local read "stop"() -> (w194:bool)
          n152 = Or(x=w194, y=w192) -> (x .or. y?=w189:bool)
          n153 = call <vilib>:"Application Directory.vi"() -> ()  [unwired: 1 out]
        }
      }
      event "删除标注": Value Change {
        w272 = T5."Disabled and Grayed Out" ("禁用")
        n154 = event-data() -> ()  [unwired: 1 in, 6 out]
        n155 = call "用户输入2"() -> ("框号"=w273:dbl, "确定"=w274:bool)  [unwired: 17 in, 1 out]
        n156 = property on="生成报告" class="Bool"("DisabledEnum"=T5."Enabled" ("禁用")) -> ()  [unwired: 2 in, 2 out]
        n157 = property on="完成标注" class="Bool (严格)"("DisabledEnum"=w272) -> ()  [unwired: 2 in, 2 out]
        n158 = property on="开始标注" class="Bool"("DisabledEnum"=w272) -> ()  [unwired: 2 in, 2 out]
        n159 = case shown="真" w274 {
          tunnel: w273 -> [_ w275]
          frame False {
            # "用户取消操作"
          }
          frame True {
            n160 = stacked-sequence {
              tunnel: w275 -> [_ w282 _]
              frame #0 {
                # "1. 删除所有框"
                n161 = local read "穿透图"() -> (w276:T2)
                n162 = call "IMAQ Clear Overlay"("Image"=w276) -> ()  [unwired: 9 in, 2 out]
              }
              frame #1 {
                # "2. 删除框组中指定元素"
                n163 = local read "部位信息"() -> (w279:string[])
                n164 = local read "框组"() -> (w281:T4)
                n165 = Decrement(x=w282) -> (x-1=w278:dbl)
                n166 = Delete From Array(array=w279, index=w278) -> (array with subset deleted=w277:string[])  [unwired: 1 in, 1 out]
                n167 = Delete From Array(array=w281, index=w278) -> (array with subset deleted=w280:T4)  [unwired: 1 in, 1 out]
                n168 = local write "框组"(w280) -> ()
                n169 = local write "部位信息"(w277) -> ()
              }
              frame #2 {
                # "3. 重画所有框"
                n170 = while {
                  i -> [w295]
                  stop <- w286 stop-if-true
                  n171 = local read "框组"() -> (w290:T4)
                  n172 = local read "穿透图"() -> (w294:T2)
                  n173 = Array Size(array=w290) -> (size(s)=w291:i32)
                  n174 = Index Array(array=w290, index=w295) -> (element=w285:T6)
                  n175 = Increment(x=w295) -> (x+1=w302:i32)
                  n176 = local write "框数"(w291) -> ()
                  n177 = Greater Or Equal?(x=w302, y=w291) -> (x >= y?=w286:bool)
                  n178 = call "IMAQ Overlay ROI"("ROI Descriptor"=w285, "Image"=w294) -> ("Image Out"=w300:T2)  [unwired: 8 in, 1 out]
                  n179 = Unbundle(w285) -> ("Global Rectangle"=w292:i32[])  [unwired: 1 out]
                  n180 = Number To Decimal String(number=w302) -> (decimal integer string=w287:string)  [unwired: 1 in]
                  n181 = Index Array(array=w292, index=0 ("索引")) -> (element=w297:i32)
                  n182 = Index Array(array=w292, index=1 ("索引")) -> (element=w298:i32)
                  n183 = local read "自定义字体"() -> (w284:T3)
                  n184 = Concatenate Strings(w287, "#" ("字符串")) -> (w283:string)
                  n185 = Bundle(w297, w298) -> (w288:cluster{i32, i32})  [unwired: 1 in]
                  n186 = call "IMAQ Overlay Text"("Text Color (black)"=u32 16711680, "Font, Size & Style"=w284, "String"=w283, "Origin"=w288, "Image"=w300) -> ("Image Out"=w293:T2)  [unwired: 5 in, 1 out]
                  n187 = local write "穿透图"(w293) -> ()
                }
              }
            }
          }
        }
      }
      event "查看评定结果": Value Change {
        w311 = T5."Disabled and Grayed Out" ("禁用")
        # "只读穿透图的图像处理方法"
        # "查看指定框的详细信息，包括灰度和面积阈值分割后的结果，提取到的长宽面积等信息"
        n188 = event-data() -> ()  [unwired: 1 in, 6 out]
        n189 = property on="完成标注" class="Bool (严格)"("DisabledEnum"=w311) -> ()  [unwired: 2 in, 2 out]
        n190 = local read "判定为筋条的长宽比阈值"() -> (w306:i32)
        n191 = property on="开始标注" class="Bool"("DisabledEnum"=w311) -> ()  [unwired: 2 in, 2 out]
        n192 = local read "计入缺陷的面积阈值"() -> (w309:i32)
        n193 = local read "临界面积百分比值"() -> (w313:dbl)
        n194 = local read "计入缺陷的Z值阈值"() -> (w307:i32)
        n195 = local read "图像Y向分辨率（mm/像素）"() -> (w304:dbl)
        n196 = local read "图像X向分辨率（mm/像素）"() -> (w305:dbl)
        n197 = local read "缺陷灰度阈值"() -> (w308:dbl)
        n198 = local read "临界Z值"() -> (w314:i32)
        n199 = local read "部位信息"() -> (w316:string[])
        n200 = local read "穿透图"() -> (w303:T2)
        n201 = local read "框组"() -> (w315:T4)
        n202 = call "子VI-查看某框.vi"("输入框号"=0.0 ("框号"), "框组"=w315, "判定为筋条的长宽比阈值"=w306, "临界Z值"=w314, "缺陷灰度阈值"=w308, "临界面积百分比值"=w313, "计入缺陷的面积阈值"=w309, "计入缺陷的Z值阈值"=w307, 8:w303, "部位信息"=w316, "长度方向分辨率（Y方向，mm/像素）"=w304, "宽度方向分辨率（X方向，mm/像素）"=w305) -> ("全部检测结果"=→"全部检测结果":string[][])  [unwired: 15 in]
      }
      event "生成报告": Value Change {
        w329 = T5."Disabled and Grayed Out" ("禁用")
        # "相当于“查看标注”一栏中的操作做循环，遍历所有框，\n将输出结果叠加为数组，作为最终结果输出并导入word"
        n203 = event-data() -> ()  [unwired: 1 in, 6 out]
        n204 = local read "图像X向分辨率（mm/像素）"() -> (w319:dbl)
        n205 = call "报告模式选择"() -> ("深度学习方法"=w328:bool, "自动检测结果"=w331:bool, "手动框选结果"=w332:bool, "确定"=w330:bool)  [unwired: 15 in, 1 out]
        n206 = local read "图像Y向分辨率（mm/像素）"() -> (w318:dbl)
        n207 = local read "计入缺陷的面积阈值"() -> (w325:i32)
        n208 = Build Array(w332, w331, w328) -> (w334:bool[])
        n209 = local read "临界面积百分比值"() -> (w336:dbl)
        n210 = local read "判定为筋条的长宽比阈值"() -> (w324:i32)
        n211 = local read "计入缺陷的Z值阈值"() -> (w326:i32)
        n212 = local read "缺陷灰度阈值"() -> (w335:dbl)
        n213 = Boolean Array To Number(Boolean array=w334) -> (number=w333:u32)
        n214 = local read "部位信息"() -> (w339:string[])
        n215 = local read "框组"() -> (w338:T4)
        n216 = property on="删除标注" class="Bool (严格)"("DisabledEnum"=w329) -> ()  [unwired: 2 in, 2 out]
        n217 = property on="完成标注" class="Bool (严格)"("DisabledEnum"=w329) -> ()  [unwired: 2 in, 2 out]
        n218 = property on="开始标注" class="Bool"("DisabledEnum"=w329) -> ()  [unwired: 2 in, 2 out]
        n219 = Bundle("图像X向分辨率（mm/像素）"=w319, "图像Y向分辨率（mm/像素）"=w318) -> (w317:T1)  [unwired: 1 in]
        "XY向分辨率" <- w317
        n220 = Initialize Array(i8 0 ("元素"), 0 ("维数大小")) -> (w320:i8[])
        n221 = local read "穿透图"() -> (w323:T2)
        n222 = local read "临界Z值"() -> (w337:i32)
        n223 = case shown="真" w330 {
          tunnel: w339 -> [_ w357]
          tunnel: w338 -> [_ w356]
          tunnel: w337 -> [_ w355]
          tunnel: w336 -> [_ w354]
          tunnel: string[][] [] ("分层类检测结果合并 2") -> [_ w353]
          tunnel: w335 -> [_ w352]
          tunnel: w333 -> [_ w351]
          tunnel: w326 -> [_ w348]
          tunnel: w325 -> [_ w347]
          tunnel: w324 -> [_ w345]
          tunnel: w323 -> [_ w344]
          tunnel: w320 -> [_ w343]
          tunnel: w317 -> [_ w341]
          frame False {
          }
          frame True {
            n224 = case shown="0, 默认" w351 {
              tunnel: [w373 w416 w462 w471] -> w358
              tunnel: w357 -> [w375 w422 w466 _]
              tunnel: w356 -> [w376 w421 w465 _]
              tunnel: w355 -> [w378 w418 w464 w476]
              tunnel: w354 -> [w379 w419 w463 w473]
              tunnel: w353 -> [w380 w417 w461 w478]
              tunnel: w352 -> [w377 w420 w457 w475]
              tunnel: w348 -> [w371 w415 w458 w472]
              tunnel: w347 -> [w370 w414 w459 w474]
              tunnel: w345 -> [w369 w413 w456 w470]
              tunnel: w344 -> [w368 w412 w455 _]
              tunnel: w343 -> [w367 w411 _ _]
              tunnel: [w366 w410 i32[] [] i32[] []] -> w342
              tunnel: w341 -> [w365 w409 w453 _]
              frame 0, Default {
                # "默认手动框选结果"
                n225 = local read "框数"() -> (w374:dbl)
                n226 = for {
                  N: w374 -> [_]
                  shift-right: [w404] -> w373
                  shift-left: w380 -> [w403]
                  tunnel: w375 -> [w402]
                  tunnel: w376 -> [w401]
                  tunnel: w379 -> [w400]
                  tunnel: w377 -> [w395]
                  tunnel: w378 -> [w399]
                  tunnel: w371 -> [w396]
                  tunnel: w370 -> [w397]
                  tunnel: w369 -> [w394]
                  tunnel: w368 -> [w393]
                  shift-right: [w390] -> w366
                  shift-left: w367 -> [w391]
                  tunnel: w365 -> [w387]
                  i -> [w388]
                  # "2023.8.9\n生成到报告中的框号需要递增，\nflag=1 表示该框有缺陷，\n框号值递增1，否则框号值不变"
                  n227 = local read "框号-更新后按顺序的值"() -> (w384:i32)
                  n228 = Increment(x=w388) -> (x+1=w389:i32)
                  n229 = local read "框号-更新后按顺序的值"() -> (w381:i32)
                  n230 = call "子VI-查看某框-不显示界面.vi"("框号"=w389, "框组"=w401, "计入缺陷的Z值阈值"=w396, "临界Z值"=w399, "计入缺陷的面积阈值"=w397, "临界面积百分比值"=w400, "XY向分辨率"=w387, "缺陷灰度阈值"=w395, 8:w393, "部位信息"=w402, "判定为筋条的长宽比阈值"=w394, "框号-更新后按顺序的值"=w384) -> ("全部检测结果"=w398:string[][], "flag标记簇"=w392:cluster{"框号":dbl, "数值":i32})  [unwired: 14 in]
                  n231 = Unbundle(w392) -> ("数值"=w386:i32)  [unwired: 1 out]
                  n232 = Equal?(x=w386, y=1) -> (x = y?=w383:bool)
                  n233 = case shown="真" w383 {
                    tunnel: [w405 w406] -> w382
                    tunnel: w381 -> [w405 w407]
                    frame False {
                    }
                    frame True {
                      n234 = Increment(x=w407) -> (x+1=w406:i32)
                    }
                  }
                  n235 = Build Array (concatenate)(w391, w386) -> (w390:i32[])
                  n236 = Build Array (concatenate)(w403, w398) -> (w404:string[][])
                  n237 = local write "框号-更新后按顺序的值"(w382) -> ()
                }
                "报告模式" <- "手动框选"
                "框号-更新后按顺序的值" <- 1 ("框号-更新后按顺序的值")
              }
              frame 1 {
                n238 = local write "报告模式"("手动框选") -> ()
                n239 = local write "框号-更新后按顺序的值"(1 ("框号-更新后按顺序的值")) -> ()
                n240 = local read "框数"() -> (w423:dbl)
                n241 = for {
                  N: w423 -> [_]
                  shift-right: [w448] -> w416
                  shift-left: w417 -> [w447]
                  tunnel: w422 -> [w446]
                  tunnel: w421 -> [w445]
                  tunnel: w420 -> [w439]
                  tunnel: w419 -> [w444]
                  tunnel: w418 -> [w443]
                  tunnel: w415 -> [w440]
                  tunnel: w414 -> [w441]
                  tunnel: w413 -> [w438]
                  tunnel: w412 -> [w437]
                  shift-right: [w435] -> w410
                  shift-left: w411 -> [w434]
                  tunnel: w409 -> [w431]
                  i -> [w432]
                  # "2023.8.9\n生成到报告中的框号需要递增，\nflag=1 表示该框有缺陷，\n框号值递增1，否则框号值不变"
                  n242 = local read "框号-更新后按顺序的值"() -> (w427:i32)
                  n243 = local read "框号-更新后按顺序的值"() -> (w425:i32)
                  n244 = Increment(x=w432) -> (x+1=w433:i32)
                  n245 = call "子VI-查看某框-不显示界面.vi"("框号"=w433, "框组"=w445, "计入缺陷的Z值阈值"=w440, "临界Z值"=w443, "计入缺陷的面积阈值"=w441, "临界面积百分比值"=w444, "XY向分辨率"=w431, "缺陷灰度阈值"=w439, 8:w437, "部位信息"=w446, "判定为筋条的长宽比阈值"=w438, "框号-更新后按顺序的值"=w427) -> ("全部检测结果"=w442:string[][], "flag标记簇"=w436:cluster{"框号":dbl, "数值":i32})  [unwired: 14 in]
                  n246 = Unbundle(w436) -> ("数值"=w430:i32)  [unwired: 1 out]
                  n247 = Equal?(x=w430, y=1) -> (x = y?=w429:bool)
                  n248 = case shown="假" w429 {
                    tunnel: [w449 w450] -> w426
                    tunnel: w425 -> [w449 w451]
                    frame False {
                    }
                    frame True {
                      n249 = Increment(x=w451) -> (x+1=w450:i32)
                    }
                  }
                  n250 = Build Array (concatenate)(w447, w442) -> (w448:string[][])
                  n251 = Build Array (concatenate)(w434, w430) -> (w435:i32[])
                  n252 = local write "框号-更新后按顺序的值"(w426) -> ()
                }
              }
              frame 2 {
                w452 = 0.0 ("框号")
                n253 = local write "报告模式"("自动检测") -> ()
                n254 = call "子VI-查看某框-不显示界面.vi"("框号"=w452, "框组"=w465, "计入缺陷的Z值阈值"=w458, "临界Z值"=w464, "计入缺陷的面积阈值"=w459, "临界面积百分比值"=w463, "XY向分辨率"=w453, "缺陷灰度阈值"=w457, 8:w455, "部位信息"=w466, "判定为筋条的长宽比阈值"=w456, "框号-更新后按顺序的值"=w452) -> ("全部检测结果"=w460:string[][])  [unwired: 14 in, 1 out]
                n255 = Build Array (concatenate)(w461, w460) -> (w462:string[][])
              }
              frame 4 {
                # "深度学习方法自动检测demo"
                n256 = local read "穿透图原始路径"() -> (w469:path)
                n257 = local write "报告模式"("深度学习自动检测" ("报告模式")) -> ()
                n258 = call "子VI-深度学习自动检测.vi"("临界Z值"=w476, "判定为筋条的长宽比阈值"=w470, "临界面积百分比值"=w473, "缺陷灰度阈值"=w475, "计入缺陷的面积阈值"=w474, "穿透图原始路径"=w469, "计入缺陷的Z值阈值"=w472) -> ("全部检测结果"=w477:string[][])  [unwired: 8 in]
                n259 = Build Array (concatenate)(w477, w478) -> (w471:string[][])
              }
            }
            "flag数组" <- w342
            n260 = flat-sequence {
              tunnel: w358 -> [w483]
              tunnel: [w482] -> w346
              tunnel: [w484] -> w363
              tunnel: w346 -> [w484]
              tunnel: w363 -> [w538]
              tunnel: [w538] -> w362
              tunnel: w362 -> [w544]
              tunnel: [w544] -> w361
              tunnel: [w540] -> w350
              tunnel: [w539] -> w349
              tunnel: [w572] -> w360
              tunnel: [w571] -> w359
              tunnel: w361 -> [w565]
              tunnel: w350 -> [w562]
              tunnel: w349 -> [w561]
              tunnel: w359 -> [w590]
              tunnel: w360 -> [w591]
              frame #0 {
                # "2023.7.21\n增加手动修改评定结果子vi\n手动修改类型点击确认再判定和生成报告"
                n261 = local read "临界面积百分比值"() -> (w481:dbl)
                n262 = call "子VI-修改评定结果.vi"("全部检测结果"=w483, "临界面积百分比值"=w481) -> ("全部检测结果合并输出"=w482:string[][])  [unwired: 9 in]
                "框号-报告图中按顺序的值" <- 1
              }
              frame #1 {
                n263 = while {
                  tunnel: [w496] -> _
                  i -> [w486]
                  stop <- w496 stop-if-true
                  # "2023.8.8\n分析框组，如果没有结果，\n不绘制在报告图上"
                  # "生成绘制了ROI的图像\n可以用于后续的图片导出保存"
                  n264 = local read "框组"() -> (w497:T4)
                  n265 = local read "ROImask"() -> (w490:T2)
                  n266 = local read "flag数组"() -> (w493:i8[])
                  n267 = local read "穿透图"() -> (w487:T2)
                  n268 = Array Size(array=w497) -> (size(s)=w498:i32)
                  n269 = Index Array(array=w497, index=w486) -> (element=w489:T6)
                  n270 = Increment(x=w486) -> (x+1=w485:i32)
                  n271 = Index Array(array=w493, index=w486) -> (element=w492:i8)
                  n272 = Greater Or Equal?(x=w485, y=w498) -> (x >= y?=w496:bool)
                  n273 = Equal?(x=w492, y=i8 1) -> (x = y?=w488:bool)
                  n274 = case shown="真" w488 {
                    tunnel: [w500 w518] -> w495
                    tunnel: [errorcluster {"status"=FALSE, "code"=0, "source"=""} ("error out") w506] -> w494
                    tunnel: w490 -> [w500 w505]
                    tunnel: w489 -> [_ w504]
                    tunnel: w487 -> [_ w503]
                    frame False {
                    }
                    frame True {
                      w524 = 1 items=["White", "Black", "Inverted", "Black on White", "White on Black"] ("Color")
                      w526 = u16 2 items=["Frame", "Paint", "Invert Frame", "Invert Paint"] ("Draw Mode")
                      w521 = u16 1 items=["Line", "Rectangle", "Oval"] ("Shape to draw")
                      n275 = Unbundle By Name(w504) -> ("Global Rectangle"=w513:i32[])
                      n276 = local read "框号-报告图中按顺序的值"() -> (w502:i32)
                      n277 = Index Array(array=w513, index=2 ("索引")) -> (element=w512:i32)
                      n278 = Index Array(array=w513, index=0 ("索引")) -> (element=w509:i32)
                      n279 = Index Array(array=w513, index=3 ("索引")) -> (element=w511:i32)
                      n280 = Index Array(array=w513, index=1 ("索引")) -> (element=w508:i32)
                      n281 = Build Array(w509, w508, w512, w511) -> (w510:i32[])
                      n282 = Increment(x=w502) -> (x+1=w501:i32)
                      n283 = call "IMAQ Draw"("Draw Mode"=w526, "Shape to draw"=w521, "Coordinates"=w510, "Image Src"=w503) -> ("Image Dst Out"=w525:T2)  [unwired: 6 in, 1 out]
                      n284 = Number To Decimal String(number=w502) -> (decimal integer string=w522:string)  [unwired: 1 in]
                      n285 = local write "框号-报告图中按顺序的值"(w501) -> ()
                      n286 = local read "自定义字体"() -> (w519:T3)
                      n287 = Concatenate Strings(w522, "#" ("字符串")) -> (w520:string)
                      n288 = Build Array(w509, w508) -> (w507:i32[])
                      n289 = call "IMAQ Draw Text"("String"=w520, "Insertion Point"=w507, "Color"=w524, "Font, Size & Style"=w519, "Image Dst"=w505, "Image Src"=w525) -> ("error out"=w506:errorcluster, "Image Dst Out"=w518:T2)  [unwired: 2 in, 2 out]
                      n290 = local write "ROImask"(w518) -> ()
                    }
                  }
                  "ROImask" <- w495
                  n291 = case shown="错误" w494 {
                    frame No Error {
                    }
                    frame Error {
                      n292 = One Button Dialog(message="失败！无法保存图片到报告" ("消息")) -> ()  [unwired: 1 in, 1 out]
                    }
                  }
                }
              }
              frame #2 {
                n293 = local read "穿透图原始路径"() -> (w537:path)
                n294 = local read "ROImask"() -> (w529:T2)
                n295 = Path To String(path=w537) -> (string=w534:string)
                n296 = String Length(string=w534) -> (length=w535:i32)
                n297 = Subtract(x=w535, y=4) -> (x-y=w536:i32)
                n298 = Replace Substring(3:w536, 4:"_标注后.png" ("字符串"), 5:w534) -> (1:w533:string)  [unwired: 1 in, 1 out]
                n299 = String To Path(string=w533) -> (path=w528:path)
                "标注后的图片路径" <- w528
                n300 = call-poly "IMAQ Write File 2"("Image Quality"=u32 1000, "File Path"=w528, "Image"=w529) -> ()  [unwired: 7 in, 2 out]
              }
              frame #3 {
                # "最终检测结果全部合并 导入word中"
                n301 = call <vilib>:"Application Directory.vi"() -> ("Application Directory"=w543:path)
                n302 = Build Path(base path=w543, name or relative path="report-template.docx") -> (appended path=w541:path)
                n303 = call <vilib>:"Create Report.vi"("window state (normal)"=T8."maximized", "report type"=Report_Type."Word", "template (empty)"=w541) -> ("report out"=w540:refnum<class "NI_report.lvclass">, "error out"=w539:errorcluster)  [unwired: 11 in]
              }
              frame #4 {
                n304 = local read "报告模式"() -> (w563:string)
                n305 = local read "质量等级"() -> (w559:string)
                n306 = Get Date/Time String(date format (0)=enum16{"short", "long", "abbreviated"}."long" ("日期格式(0)")) -> (date string=w569:string, time string=w570:string)  [unwired: 2 in]
                n307 = call-poly <vilib>:"Append Report Text.vi"("report in"=w562, "MS Office parameters"=T12 {"position (excel)"={"row"=0, "column"=0}, "name (excel)"="", "bookmark (word)"="mode"}, "text"=w563, "error in (no error)"=w561) -> ("report out"=w558:refnum<class "NI_report.lvclass">, "error out"=w557:errorcluster)  [unwired: 8 in, 2 out]
                n308 = Concatenate Strings(w569, w570) -> (w568:string)
                n309 = local read "标注后的图片路径"() -> (w552:path)
                n310 = call-poly <vilib>:"Append Report Text.vi"("report in"=w558, "MS Office parameters"=T12 {"position (excel)"={"row"=0, "column"=0}, "name (excel)"="", "bookmark (word)"="class"}, "text"=w559, "error in (no error)"=w557) -> ("report out"=w555:refnum<class "NI_report.lvclass">, "error out"=w556:errorcluster)  [unwired: 8 in, 2 out]
                n311 = call-poly <vilib>:"Append Report Text.vi"("report in"=w555, "MS Office parameters"=T12 {"position (excel)"={"row"=0, "column"=0}, "name (excel)"="", "bookmark (word)"="time"}, "text"=w568, "error in (no error)"=w556) -> ("report out"=w549:refnum<class "NI_report.lvclass">, "error out"=w550:errorcluster)  [unwired: 8 in, 2 out]
                n312 = call-poly <vilib>:"Append Image to Report.vi"("report in"=w549, "alignment (default)"=HTML_Report_Image_Alignment."MIDDLE", "MS Office parameters"=T11 {"position (Excel)"={"row"=0, "column"=0}, "name (Excel)"="", "bookmark (Word)"="image"}, "path or URL of image"=w552) -> ("report out"=w548:refnum<class "NI_report.lvclass">, "error out"=w551:errorcluster)  [unwired: 8 in, 2 out]
                n313 = call <vilib>:"Word Easy Text.vi"("report in"=w548, "text"="检测结果：", "alignment (left)"=enum16{"Left", "Centered", "Right", "Justify"}."Left", "font"=T13 {"font name"="", "font size"=0.0, "bold"=0, "italic"=0, "underline"=0, "strike through"=0, "font color"=16777216}, "error in (no error)"=w550) -> ("report out"=w547:refnum<class "NI_report.lvclass">, "error out"=w574:errorcluster)  [unwired: 8 in, 1 out]
                n314 = call-poly <vilib>:"Word Easy Table.vi"("report in"=w547, "column headers"=string[] ["框号", "X/mm", "Y/mm", "长/mm", "宽/mm", "面积/mm2", "Z值/mm", "部位", "类型", "合格性"], "data"=w565, "error in (no error)"=w574) -> ("report out"=w572:refnum<class "NI_report.lvclass">, "error out"=w571:errorcluster)  [unwired: 9 in, 1 out]
                n315 = case shown="错误" w551 {
                  frame No Error {
                  }
                  frame Error {
                    n316 = One Button Dialog(message="图片导入word\n发生错误！" ("消息")) -> ()  [unwired: 1 in, 1 out]
                  }
                }
              }
              frame #5 {
                n317 = local read "穿透图原始路径"() -> (w583:path)
                n318 = local read "报告模式"() -> (w581:string)
                n319 = Path To String(path=w583) -> (string=w587:string)
                n320 = String Length(string=w587) -> (length=w588:i32)
                n321 = Subtract(x=w588, y=4) -> (x-y=w589:i32)
                n322 = Concatenate Strings("_" ("字符串"), w581, ".docx" ("字符串")) -> (w579:string)
                n323 = Replace Substring(3:w589, 4:w579, 5:w587) -> (1:w586:string)  [unwired: 1 in, 1 out]
                n324 = String To Path(string=w586) -> (path=w584:path)
                "添加的路径" <- w584
                n325 = call-dynamic "Save Report to File.vi"("report in"=w591, "report file path"=w584, "prompt to replace? (F)"=TRUE, "error in (no error)"=w590) -> ("report out"=w595:refnum<class "NI_report.lvclass">, "error out"=w594:errorcluster)  [unwired: 10 in]
                n326 = call <vilib>:"Word Bring to Front.vi"("report in"=w595, "window state (maximized)"=enum16{"maximized", "minimized", "normal"}."normal", "error in (no error)"=w594) -> ()  [unwired: 11 in, 2 out]
              }
              frame #6 {
                n327 = local write "全部检测结果合并"(string[][] [] ("弥散类检测结果合并")) -> ()
                n328 = One Button Dialog(message="完成评定并退出程序！\n请查看word报告" ("消息")) -> ()  [unwired: 1 in, 1 out]
              }
            }
          }
        }
      }
      event "stop": Value Change {
        # "退出软件"
        n329 = event-data() -> ("NewVal"=w601:bool)  [unwired: 1 in, 4 out]
        n330 = Two Button Dialog(message="是否关闭本软件？" ("消息")) -> (T button?=w602:bool)  [unwired: 2 in]
        n331 = And(x=w601, y=w602) -> (x .and. y?=w600:bool)
        n332 = case shown="真" w600 {
          frame False {
          }
          frame True {
            n333 = local read "穿透图"() -> (w604:T2)
            n334 = call "Imaq Dispose"("All Images? (No)"=TRUE, "Image"=w604) -> ()  [unwired: 4 in, 1 out]
            n335 = disable-structure shown="RUN_TIME_ENGINE==True" {
              frame condition #0 {
                n336 = Quit LabVIEW() -> ()  [unwired: 1 in]
              }
              frame condition #1 (active) {
                n337 = Stop() -> ()  [unwired: 1 in]
              }
            }
          }
        }
      }
    }
  }
  n338 = disable-structure shown="启用" {
    frame Disabled {
      n339 = while {
        stop <- FALSE stop-if-true
        n340 = local read "查看评定结果"() -> (w607:bool)
        n341 = local read "删除标注"() -> (w608:bool)
        n342 = Or(x=w608, y=w607) -> (x .or. y?=w609:bool)
        n343 = local write "开始标注"(w609) -> ()
        n344 = Wait Until Next ms Multiple(millisecond multiple=u32 50 ("毫秒倍数")) -> ()  [unwired: 1 out]
      }
    }
    frame Enabled {
    }
  }
  n345 = disable-structure shown="启用" {
    frame Disabled {
    }
    frame Enabled {
    }
  }
  "临界面积百分比值" <- w15
  "缺陷灰度阈值" <- w16
